vi "niFPGA Relay_m.vi"   [LabVIEW 2017]
doc: "Switches between the <B>output when on</B> and <B>output when off</B> inputs. When the relay is on, it remains on until <B>input</B> is less than <B>switch off point</B>. When the relay is off, it remains off until <B>input</B> is greater than <B>switch on point</B>. The relay is off by default. The data type you wire to <B>input</B> determines the <B>output</B> data type."
uses:
  <vilib>/rvi/Analysis/common/FxpNativeNode/niFpgaFxpNative.xnode
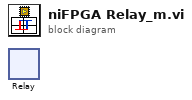
[diagram p0: block diagram]
diagram:
  n1 = xnode ("Relay")() -> ()  [unwired: 6 in, 1 out]
